vi "Read StdOut Log.vi"(8 "error in (no error)":errorcluster, 11 "Optimiser Cell in":refnum<class "Optimiser Cell.lvclass">) -> (0 "error out":errorcluster, 2 "StdOut Log":refnum<class "Log.lvclass">, 3 "Optimiser Cell out":refnum<class "Optimiser Cell.lvclass">)   [LabVIEW 2020, in "CIRCUS_uServices.lvlib" / "Run Utilities.lvlib" / "Optimiser Cell.lvclass"]
uses:
  Optimiser Cell.lvclass
  Optimiser Cell.lvclass/Optimiser Cell.ctl
  TALOS/TALOS_PPL.lvlibp/Classes/Log/Log.lvclass
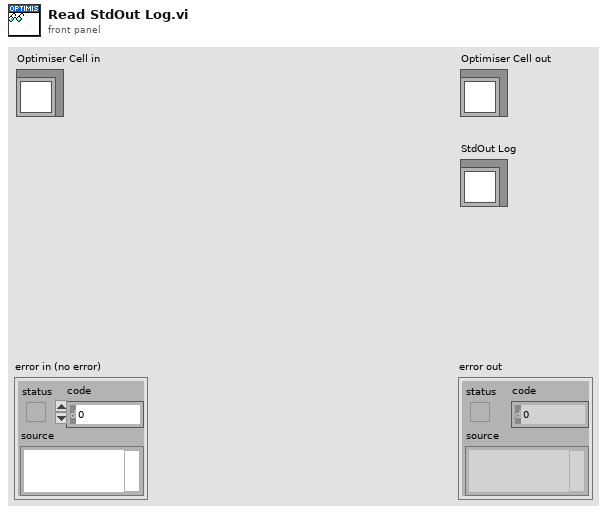
[diagram p1: front panel]
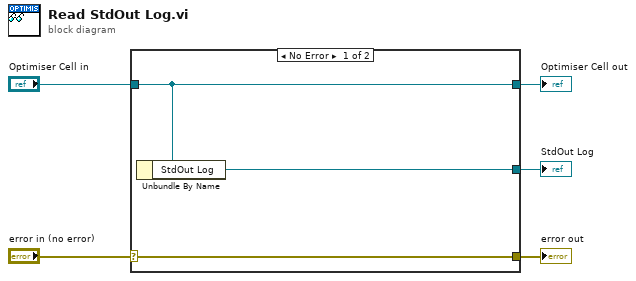
[diagram p0: block diagram]
diagram:
  n1 = case shown="No Error" "error in (no error)" {
    selector: "error in (no error)" -> [w8 w9]
    tunnel: [w8 w9] -> w4
    tunnel: [w7 w10] -> w2
    tunnel: "Optimiser Cell in" -> [w7 w10]
    tunnel: [w6 _] -> w1
    frame No Error {
      n2 = Unbundle By Name(w7) -> ("StdOut Log"=w6:refnum<class "Log.lvclass">)
    }
    frame Error {
    }
  }
  "error out" <- w4
  "Optimiser Cell out" <- w2
  "StdOut Log" <- w1
